vi "Set value by Variant.vi"(8 "error in (no error)":errorcluster, 10 "Variant":variant, 11 "Numeric Column in":refnum<class "Numeric Column.lvclass">) -> (0 "error out":errorcluster, 3 "Numeric Column out":refnum<class "Numeric Column.lvclass">)   [LabVIEW 2020, in "Basic Columns.lvlib" / "Numeric Column.lvclass"]
uses:
  Numeric Column.lvclass
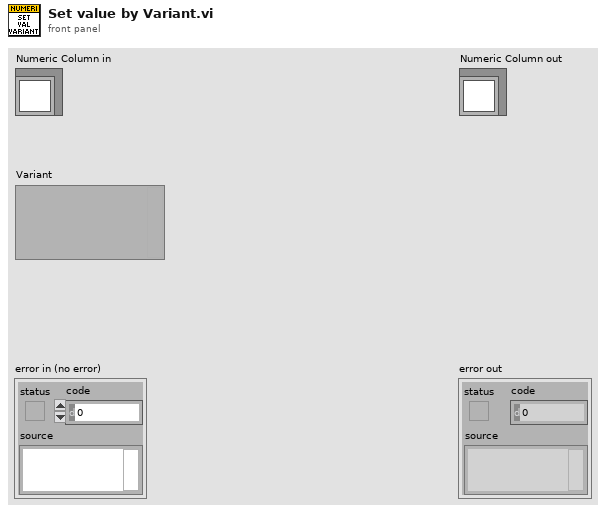
[diagram p1: front panel]
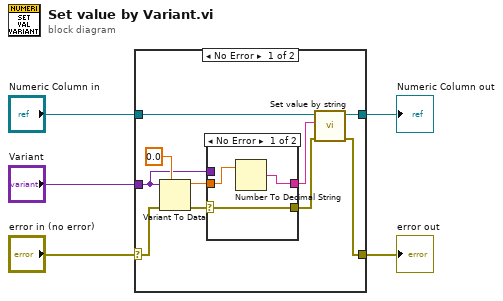
[diagram p0: block diagram]
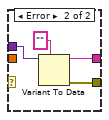
[diagram p2: hidden frame]
diagram:
  n1 = case shown="No Error" "error in (no error)" {
    selector: "error in (no error)" -> [w8 w24]
    tunnel: [w6 w24] -> w4
    tunnel: "Numeric Column in" -> [w14 w23]
    tunnel: [w15 w23] -> w2
    tunnel: "Variant" -> [w10 _]
    frame No Error {
      n2 = Variant To Data(error in=w8, type=0.0, Variant=w10) -> (data=w11:dbl, error out=w12:errorcluster)
      n3 = case shown="No Error" w12 {
        selector: w12 -> [w18 _]
        tunnel: w11 -> [w17 _]
        tunnel: w10 -> [_ w22]
        tunnel: [w16 w20] -> w9
        tunnel: [w18 w19] -> w7
        frame No Error {
          n4 = Number To Decimal String(number=w17) -> (decimal integer string=w16:string)  [unwired: 1 in]
        }
        frame Error {
          n5 = Variant To Data(type="", Variant=w22) -> (data=w20:string, error out=w19:errorcluster)  [unwired: 1 in]
        }
      }
      n6 = call-dynamic "Set value by string.vi"("error in (no error)"=w7, "Value"=w9, "Column in"=w14) -> ("error out"=w6:errorcluster, "Column out"=w15:refnum<class "Numeric Column.lvclass">)  [unwired: 7 in]
    }
    frame Error {
    }
  }
  "error out" <- w4
  "Numeric Column out" <- w2
